vi "PNG Checksum.vi"(9 "Byte":u8, 10 "Byte Array":u8[](array[numeric]), 11 "Operation":T1(ring)) -> (2 "CRC Table":u32[](array[numeric]) format="%x", 3 "CRC":u32 format="%x")   [LabVIEW 2009]
doc: "Generates a PNG compliant checksum.\n\nCode by Darin"
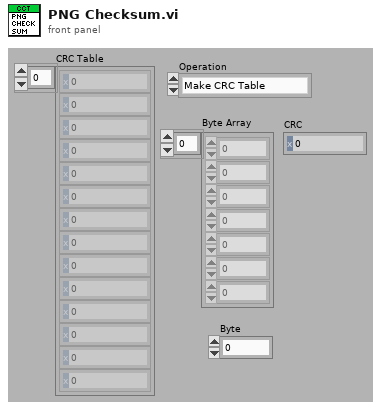
[diagram p1: front panel]
types:
  T1 = enum16{"Make CRC Table", "CRC", "Update_CRC_C", "Update_CRC_S"}
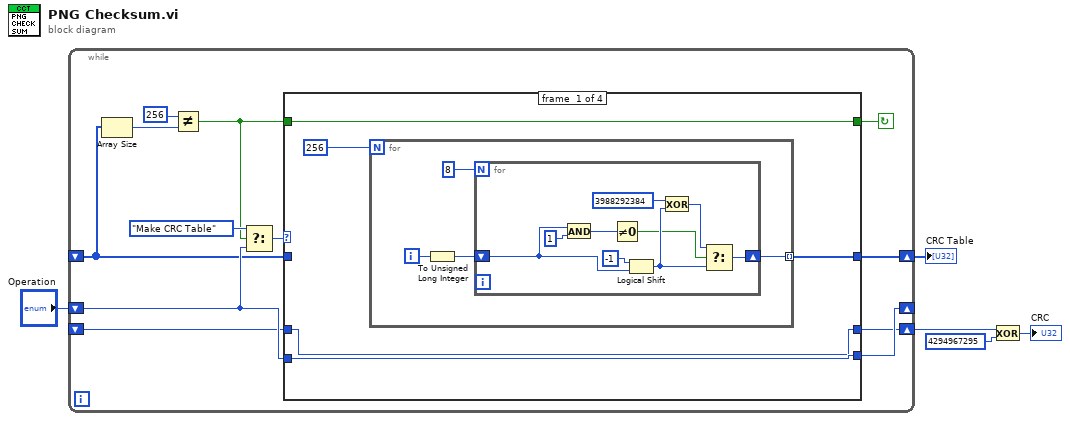
[diagram p0: block diagram]
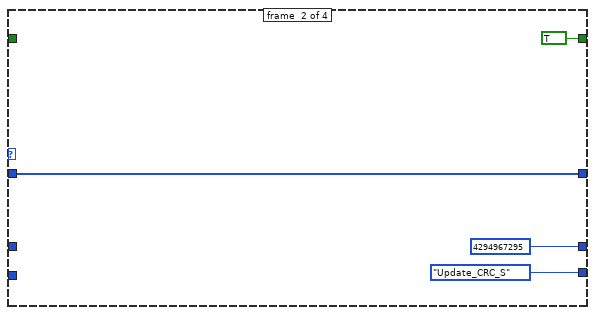
[diagram p2: hidden frame]
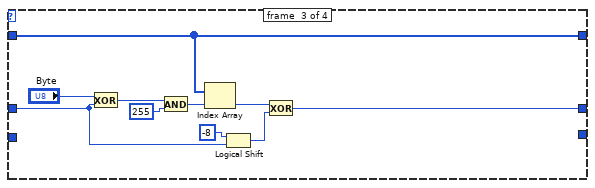
[diagram p3: hidden frame]
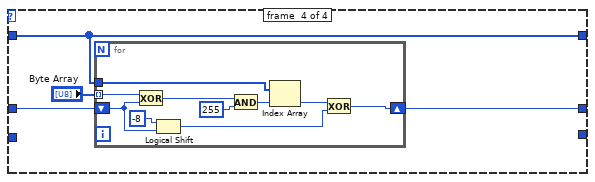
[diagram p4: hidden frame]
diagram:
  n1 = while {
    shift-right: [w11] -> w4
    shift-left: _ -> [w8]
    shift-right: [w12] -> _
    shift-left: "Operation" -> [w15]
    shift-right: [w7] -> w3
    shift-left: _ -> [w6]
    stop <- w9 continue-if-true
    n2 = Array Size(array=w8) -> (size(s)=w17:i32)
    n3 = Not Equal?(x=256, y=w17) -> (x != y?=w10:bool)
    n4 = Select(t=T1."Make CRC Table", s=w10, f=w15) -> (s? t:f=w13:T1)
    n5 = case shown="\"CRC\"" w13 {
      tunnel: w15 -> [w21 _ _ _]
      tunnel: [w21 T1."Update_CRC_S" ("Operation") _ _] -> w12
      tunnel: [w20 w39 w42 w51] -> w11
      tunnel: w10 -> [w19 _ _ _]
      tunnel: [w19 TRUE _ _] -> w9
      tunnel: w8 -> [_ w39 w42 w51]
      tunnel: [w18 u32 4294967295 w41 w50] -> w7
      tunnel: w6 -> [w18 _ w43 w53]
      frame #0 {
        n6 = for {
          N: 256 -> [_]
          tunnel: [w23] -> w20 mode=indexing
          i -> [w26]
          n7 = To Unsigned Long Integer(number=w26) -> (unsigned 32bit integer=w24:u32)
          n8 = for {
            N: 8 -> [_]
            shift-right: [w28] -> w23
            shift-left: w24 -> [w33]
            n9 = And(x=w33, y=u32 1) -> (x .and. y?=w34:u32)
            n10 = Not Equal To 0?(x=w34) -> (x != 0?=w27:bool)
            n11 = Logical Shift(y=i8 -1, x=w33) -> (x << y=w30:u32)
            n12 = Exclusive Or(1:w30, 2:u32 3988292384) -> (0:w29:u32)
            n13 = Select(t=w29, s=w27, f=w30) -> (s? t:f=w28:u32)
          }
        }
      }
      frame #1 {
      }
      frame #2 {
        n14 = Exclusive Or(1:w43, 2:"Byte") -> (0:w49:u32)
        n15 = And(x=w49, y=u8 255) -> (x .and. y?=w47:u32)
        n16 = Index Array(array=w42, index=w47) -> (element=w46:u32)
        n17 = Logical Shift(y=i8 -8, x=w43) -> (x << y=w45:u32)
        n18 = Exclusive Or(1:w45, 2:w46) -> (0:w41:u32)
      }
      frame #3 {
        n19 = for {
          shift-right: [w54] -> w50
          shift-left: w53 -> [w56]
          tunnel: "Byte Array" -> [w63] mode=indexing
          tunnel: w51 -> [w59]
          n20 = Exclusive Or(1:w56, 2:w63) -> (0:w62:u32)
          n21 = Logical Shift(y=i8 -8, x=w56) -> (x << y=w57:u32)
          n22 = And(x=w62, y=u8 255) -> (x .and. y?=w60:u32)
          n23 = Index Array(array=w59, index=w60) -> (element=w58:u32)
          n24 = Exclusive Or(1:w57, 2:w58) -> (0:w54:u32)
        }
      }
    }
  }
  "CRC Table" <- w4
  n25 = Exclusive Or(1:u32 4294967295, 2:w3) -> (0:→"CRC":u32)
